vi "AcPwrTypeFilePath.vi"(8 "error in":errorcluster, 10 "Variant":variant, 11 "Test.lvclass":refnum<class "Test.lvclass">) -> (0 "Error Out":errorcluster, 2 "PathToPluginINI":path, 3 "Test.lvclass":refnum<class "Test.lvclass">)   [LabVIEW 2018, in "Test.lvclass"]
uses:
  Test.lvclass
  Test.lvclass/Test.ctl
  Accessors/Read PluginPathArray.vi
  <vilib>/Utility/config.llb/Read Key (String).vi
  <vilib>/Utility/config.llb/NI_LVConfig.lvlib
panel:
  in  "element":string
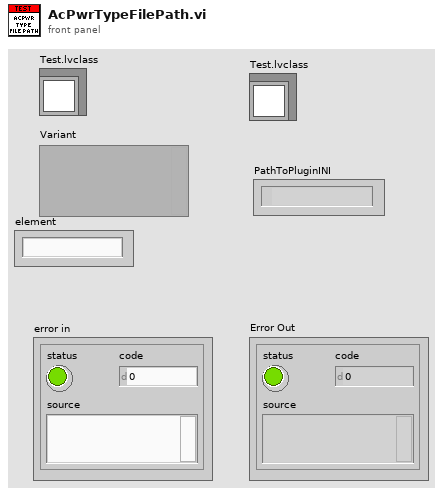
[diagram p1: front panel]
types:
  T1 = typedef "NI_LVConfig.lvlib/Config Data RefNum.ctl" = refnum<k1>
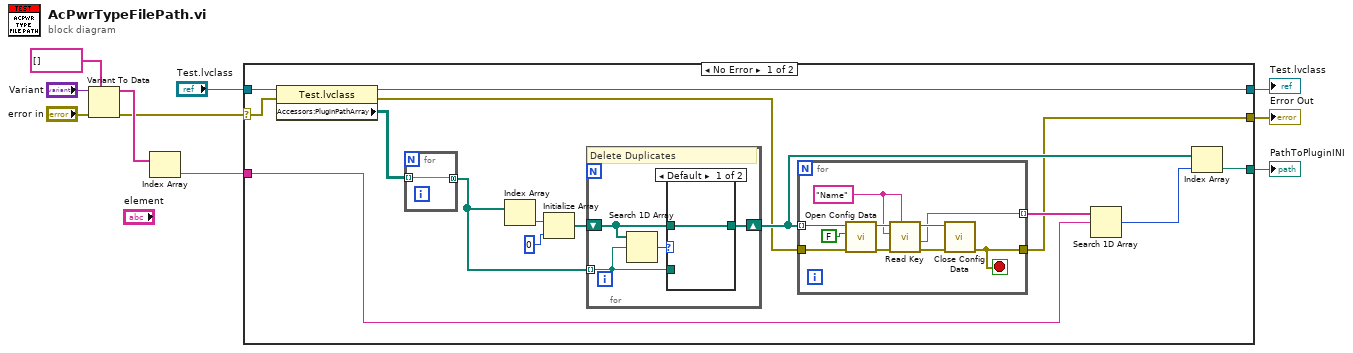
[diagram p0: block diagram]
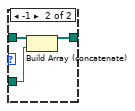
[diagram p2: hidden frame]
diagram:
  n1 = Variant To Data(error in="error in", type=string[] [], Variant="Variant") -> (data=w10:string[], error out=w8:errorcluster)
  n2 = Index Array(array=w10) -> (element=w5:string)  [unwired: 1 in]
  n3 = case shown="No Error" w8 {
    selector: w8 -> [w25 w45]
    tunnel: w5 -> [w16 _]
    tunnel: "Test.lvclass" -> [w24 w46]
    tunnel: [w23 w46] -> w3
    tunnel: [w12 w45] -> w2
    tunnel: [w13 _] -> w1
    frame No Error {
      n4 = property class="Test.lvclass"(reference=w24, error in=w25) -> (reference out=w23:refnum<class "Test.lvclass">, error out=w11:errorcluster, "Accessors:PluginPathArray"=w22:path[][])
      n5 = for {
        tunnel: w22 -> [w44] mode=indexing
        tunnel: [w44] -> w18 mode=concatenating
      }
      n6 = Index Array(array=w18) -> (element=w19:path)  [unwired: 1 in]
      n7 = Initialize Array(w19, 0 ("Dimension Size")) -> (w20:path[])
      n8 = for {
        tunnel: w18 -> [w28] mode=indexing
        shift-right: [w27] -> w15
        shift-left: w20 -> [w26]
        # "Delete Duplicates"
        n9 = Search 1D Array(1D array=w26, element=w28) -> (index of element=w29:i32)  [unwired: 1 in]
        n10 = case shown="Default" w29 {
          tunnel: w28 -> [_ w33]
          tunnel: [w30 w31] -> w27
          tunnel: w26 -> [w30 w32]
          frame Default {
          }
          frame -1 {
            n11 = Build Array (concatenate)(w32, w33) -> (w31:path[])
          }
        }
      }
      n12 = for {
        tunnel: w15 -> [w37] mode=indexing
        tunnel: [w36] -> w17 mode=indexing
        tunnel: [w35] -> w12
        tunnel: w11 -> [w34]
        stop <- w35 stop-if-true
        w38 = "Name" ("section")
        n13 = call <vilib>:"Open Config Data.vi"("error in (no error)"=w34, "create file if necessary (T)"=FALSE, "configuration file path"=w37) -> ("error out"=w42:errorcluster, "refnum"=w41:T1)  [unwired: 6 in, 1 out]
        n14 = call-poly <vilib>:"Read Key.vi"("section"=w38, "error in (no error)"=w42, "key"=w38, "refnum"=w41) -> ("error out"=w39:errorcluster, "value"=w36:string, "refnum out"=w40:T1)  [unwired: 4 in, 1 out]
        n15 = call <vilib>:"Close Config Data.vi"("error in (no error)"=w39, "refnum"=w40) -> ("error out"=w35:errorcluster)  [unwired: 8 in, 1 out]
      }
      n16 = Search 1D Array(1D array=w17, element=w16) -> (index of element=w14:i32)  [unwired: 1 in]
      n17 = Index Array(array=w15, index=w14) -> (element=w13:path)
    }
    frame Error {
    }
  }
  "Error Out" <- w2
  "Test.lvclass" <- w3
  "PathToPluginINI" <- w1
